vi "Socket Write.vi"(8 "error in (no error)":errorcluster, 9 "timeout ms (5000)":i32=5000, 10 "Bytes to write":u8[](array[numeric]), 11 "WebSocket in":refnum<class "WebSocket.lvclass">) -> (0 "error out":errorcluster, 1 "timed out?":bool, 2 "bytes written":i32, 3 "WebSocket out":refnum<class "WebSocket.lvclass">)   [LabVIEW 2021, in "WebSockets.lvlib" / "WebSocket.lvclass"]
doc: "Wrapper for the Socket Write function.\nWebSockets 2.0.1.40\nSam Sharp - MediaMongrels Ltd\nCopyright (c) 2019, MediaMongrels Ltd"
uses:
  WebSocket.lvclass
  WebSocket.lvclass/WebSocket.ctl
  Sockets/Socket/Socket.lvclass
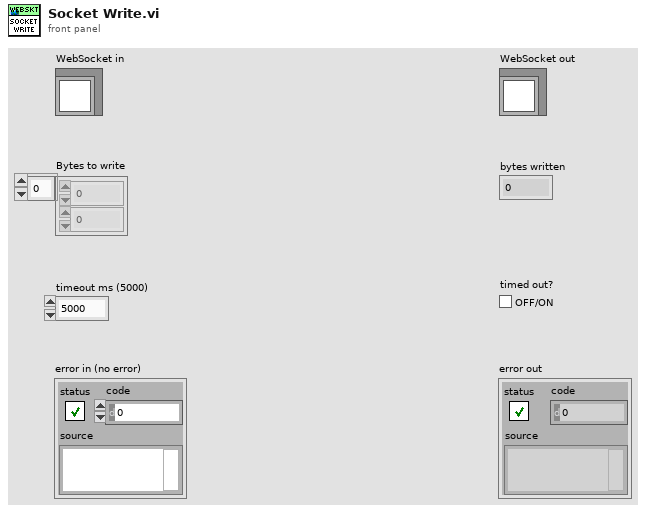
[diagram p1: front panel]
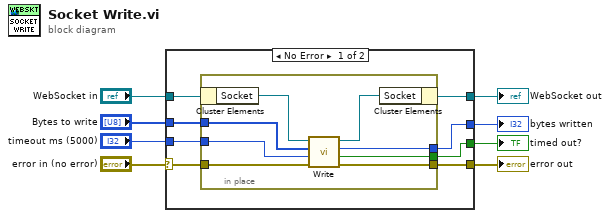
[diagram p0: block diagram]
diagram:
  n1 = case shown="No Error" "error in (no error)" {
    selector: "error in (no error)" -> [w13 w25]
    tunnel: [w10 w26] -> w6
    tunnel: "WebSocket in" -> [w16 w26]
    tunnel: "Bytes to write" -> [w15 _]
    tunnel: "timeout ms (5000)" -> [w14 _]
    tunnel: [w12 w25] -> w3
    tunnel: [w11 _] -> w2
    tunnel: [w9 _] -> w1
    frame No Error {
      n2 = in-place {
        in-place-border: w15 -> [w23]
        in-place-border: w14 -> [w22]
        in-place-border: w13 -> [w21]
        in-place-border: [w20] -> w12
        in-place-border: [w19] -> w11
        in-place-border: [w17] -> w9
        n3 = in-place-cluster #1(w16) -> ("Socket"=w24:refnum<class "Socket.lvclass">)
        n4 = call-dynamic "Write.vi"("error in (no error)"=w21, "timeout ms (25000)"=w22, "Bytes to write"=w23, "Socket in"=w24) -> ("error out"=w20:errorcluster, "timed out?"=w17:bool, "bytes written"=w19:i32, "Socket out"=w18:refnum<class "Socket.lvclass">)  [unwired: 4 in]
        n5 = in-place-cluster #1("Socket"=w18) -> (w10:refnum<class "WebSocket.lvclass">)
      }
    }
    frame Error {
    }
  }
  "error out" <- w3
  "WebSocket out" <- w6
  "bytes written" <- w2
  "timed out?" <- w1
